vi "EmergencyHallEffect (1).vi"(8 "Numeric 4":dbl, 9 "Numeric 3":dbl, 10 "Numeric 2":dbl, 11 "Numeric":dbl) -> (0 "Boolean 4":bool, 1 "Boolean 3":bool, 2 "Boolean 2":bool, 3 "Boolean":bool)   [LabVIEW 2017]
uses:
  EmergencyGLOBAL.vi
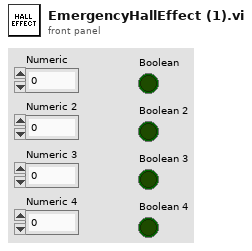
[diagram p1: front panel]
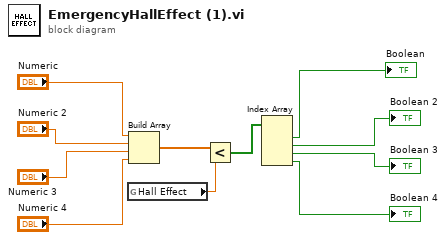
[diagram p0: block diagram]
diagram:
  n1 = global read "EmergencyGLOBAL.vi" "Hall Effect"() -> (w6:dbl)
  n2 = Build Array("Numeric", "Numeric 2", "Numeric 3", "Numeric 4") -> (w7:dbl[])
  n3 = Less?(x=w7, y=w6) -> (x < y?=w5:bool[])
  n4 = Index Array(array=w5) -> (element #1=→"Boolean":bool, element #2=→"Boolean 2":bool, element #3=→"Boolean 3":bool, element #4=→"Boolean 4":bool)  [unwired: 4 in]
